vi "Write Cylinder.vi"(10 "ActuatorCylinder":refnum<class "IActuatorCylinder.lvclass">, 11 "PressureServoActuator in":refnum<class "PressureServoActuator.lvclass">) -> (3 "PressureServoActuator out":refnum<class "PressureServoActuator.lvclass">)   [LabVIEW 2015, in "PressureServoActuator.lvclass"]
uses:
  PressureServoActuator.lvclass
  ActuatorCylinder/IActuatorCylinder/IActuatorCylinder.lvclass
  PressureServoActuator.lvclass/PressureServoActuator.ctl
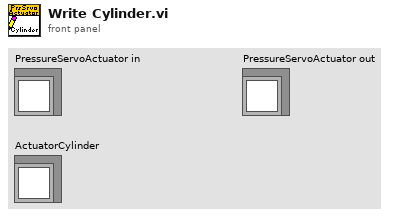
[diagram p1: front panel]
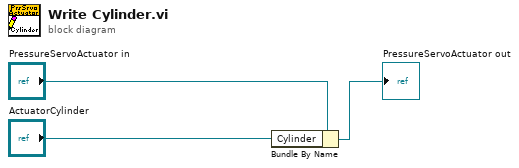
[diagram p0: block diagram]
diagram:
  n1 = Bundle By Name(cluster="PressureServoActuator in", "Cylinder"="ActuatorCylinder") -> (→"PressureServoActuator out":refnum<class "PressureServoActuator.lvclass">)
